vi "Look Up Device Properties.vi"(7 "Lookup Table":string[][](array[string]), 8 "error in (no error)":errorcluster, 9 "Peripheral ID (0)":i32, 10 "Device ID":i32) -> (0 "error out":errorcluster, 1 "Microstep Size":dbl format="%#_6f", 2 "Device Name":string, 5 "Motion Type":string)   [LabVIEW 2018, in "Zaber A Series.lvlib"]
doc: "This VI assists with looking up instrument properties in a table provided by Zaber. You can obtain the device ID and peripheral ID (if applicable) numbers from the device with the Get Device IDs VI, and use the LabVIEW Read Delimited Spreadsheet VI to load the lookup table. Given those inputs, this VI will attempt to find the device position scale factor and its name and motion type.\n\nA prepared table and a Python script for updating it are provided via Zaber's website: https://www.zaber.com/wiki/Software/ASCII_Labview_Driver\n\nNote that this VI is not optimized for speed; for efficiency, do not look up device properties inside high-speed loops.\n\nErrors are produced if the table does not have the expected format, or if the device is not found in the table."
uses:
  Zaber A Series.lvlib
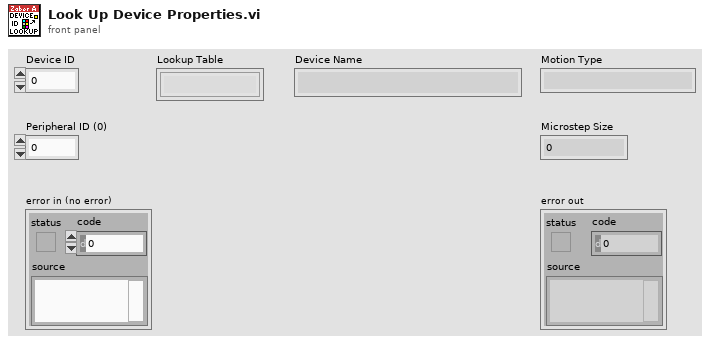
[diagram p1: front panel]
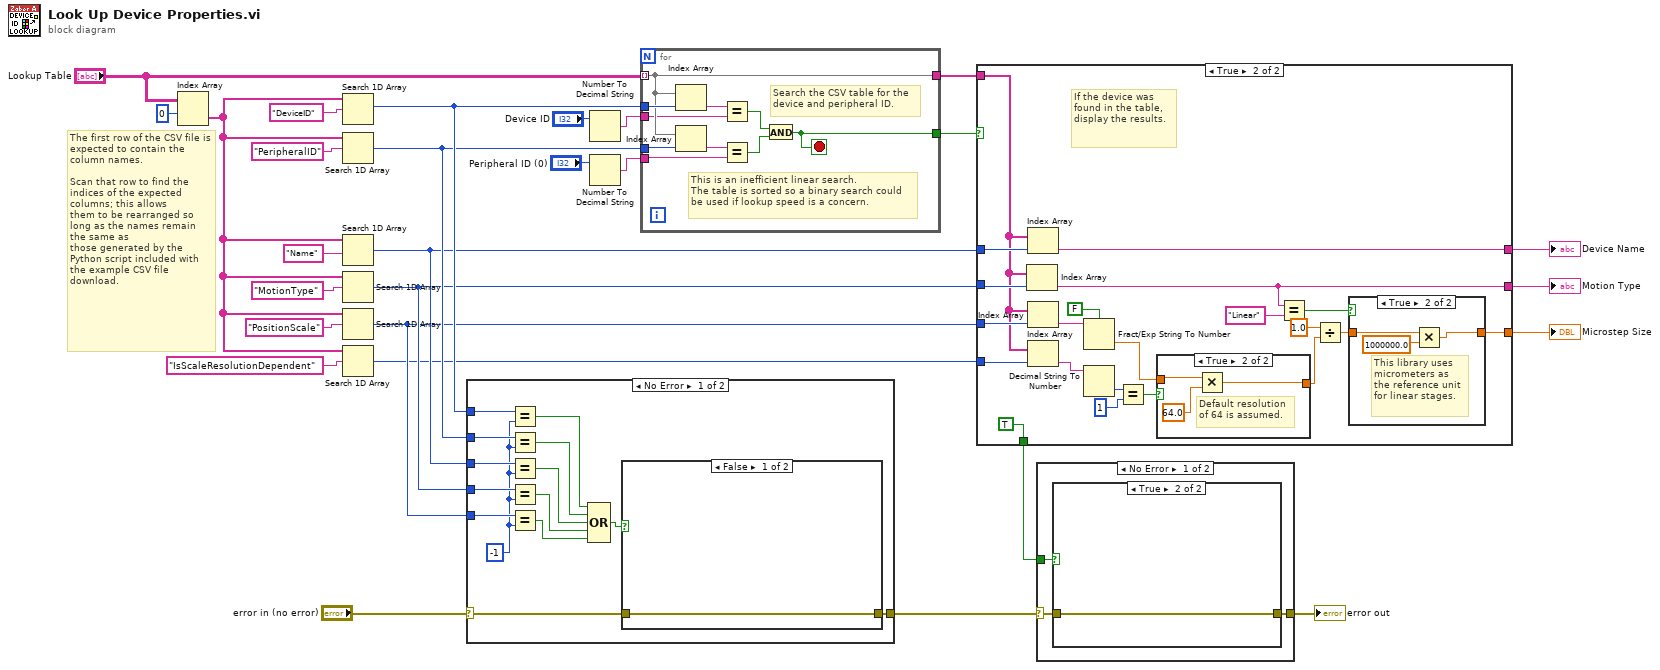
[diagram p0: block diagram]
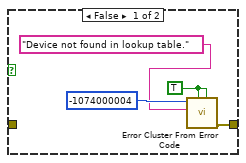
[diagram p2: hidden frame]
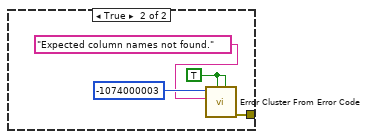
[diagram p4: hidden frame]
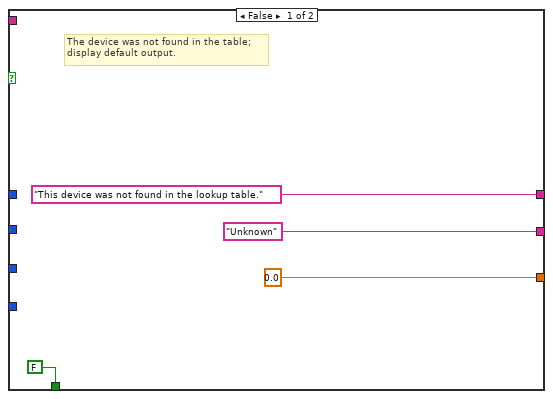
[diagram p6: hidden frame]
diagram:
  # "The first row of the CSV file is expected to contain the column names.\n\nScan that row to find the indices of the expected columns; this allows\nthem to be rearranged so long as the names remain the same as\nthose generated by the Python script included with the example CSV file download."
  n1 = Index Array(array="Lookup Table", index (row)=0) -> (element=w3:string[])  [unwired: 1 in]
  n2 = Search 1D Array(1D array=w3, element="DeviceID") -> (index of element=w16:i32)  [unwired: 1 in]
  n3 = Search 1D Array(1D array=w3, element="PeripheralID") -> (index of element=w15:i32)  [unwired: 1 in]
  n4 = Search 1D Array(1D array=w3, element="Name") -> (index of element=w14:i32)  [unwired: 1 in]
  n5 = Search 1D Array(1D array=w3, element="MotionType") -> (index of element=w13:i32)  [unwired: 1 in]
  n6 = Search 1D Array(1D array=w3, element="PositionScale") -> (index of element=w12:i32)  [unwired: 1 in]
  n7 = Search 1D Array(1D array=w3, element="IsScaleResolutionDependent") -> (index of element=w1:i32)  [unwired: 1 in]
  n8 = case shown="No Error" "error in (no error)" {
    selector: "error in (no error)" -> [w30 w48]
    tunnel: [w32 w48] -> w10
    tunnel: w16 -> [w42 _]
    tunnel: w15 -> [w41 _]
    tunnel: w14 -> [w40 _]
    tunnel: w13 -> [w39 _]
    tunnel: w12 -> [w38 _]
    frame No Error {
      w29 = -1
      n9 = Equal?(x=w42, y=w29) -> (x = y?=w37:bool)
      n10 = Equal?(x=w41, y=w29) -> (x = y?=w36:bool)
      n11 = Equal?(x=w40, y=w29) -> (x = y?=w35:bool)
      n12 = Equal?(x=w39, y=w29) -> (x = y?=w34:bool)
      n13 = Equal?(x=w38, y=w29) -> (x = y?=w33:bool)
      n14 = Compound Arithmetic op=OR(w37, w36, w35, w34, w33) -> (w31:bool)
      n15 = case shown="False" w31 {
        tunnel: [w43 w47] -> w32
        tunnel: w30 -> [w43 _]
        frame False {
        }
        frame True {
          w44 = TRUE ("show call chain? (False)")
          n16 = call <vilib>:"Error Cluster From Error Code.vi"("is warning? (False)"=w44, "show call chain? (False)"=w44, "error message (\"\")"="Expected column names not found." ("error message (\"\")"), "error code (0)"=-1074000003) -> ("error out"=w47:errorcluster)  [unwired: 5 in]
        }
      }
    }
    frame Error {
    }
  }
  n17 = Number To Decimal String(number="Device ID") -> (decimal integer string=w8:string)  [unwired: 1 in]
  n18 = Number To Decimal String(number="Peripheral ID (0)") -> (decimal integer string=w7:string)  [unwired: 1 in]
  n19 = for {
    tunnel: "Lookup Table" -> [w54] mode=indexing
    tunnel: w16 -> [w58]
    tunnel: w15 -> [w57]
    tunnel: w8 -> [w51]
    tunnel: w7 -> [w49]
    tunnel: [w54] -> w19
    tunnel: [w53] -> w23
    stop <- w53 stop-if-true
    # "This is an inefficient linear search.\nThe table is sorted so a binary search could\nbe used if lookup speed is a concern."
    # "Search the CSV table for the\ndevice and peripheral ID."
    n20 = Index Array(array=w54, index=w58) -> (element=w52:string)
    n21 = Index Array(array=w54, index=w57) -> (element=w50:string)
    n22 = Equal?(x=w52, y=w51) -> (x = y?=w56:bool)
    n23 = Equal?(x=w50, y=w49) -> (x = y?=w55:bool)
    n24 = And(x=w56, y=w55) -> (x .and. y?=w53:bool)
  }
  n25 = case shown="True" w23 {
    tunnel: ["This device was not found in the lookup table." w82] -> w22
    tunnel: ["Unknown" w75] -> w21
    tunnel: [0.0 w71] -> w20
    tunnel: w19 -> [_ w70]
    tunnel: w14 -> [_ w83]
    tunnel: w13 -> [_ w81]
    tunnel: w12 -> [_ w80]
    tunnel: [FALSE TRUE] -> w11
    tunnel: w1 -> [_ w69]
    frame False {
      # "The device was not found in the table;\ndisplay default output."
    }
    frame True {
      # "If the device was found in the table, display the results."
      n26 = Index Array(array=w70, index=w81) -> (element=w75:string)
      n27 = Index Array(array=w70, index=w83) -> (element=w82:string)
      n28 = Index Array(array=w70, index=w80) -> (element=w79:string)
      n29 = Index Array(array=w70, index=w69) -> (element=w68:string)
      n30 = Fract/Exp String To Number(use system decimal point (T)=FALSE, string=w79) -> (number=w64:dbl)  [unwired: 2 in, 1 out]
      n31 = Decimal String To Number(string=w68) -> (number=w67:i32)  [unwired: 2 in, 1 out]
      n32 = Equal?(x=w67, y=1) -> (x = y?=w65:bool)
      n33 = case shown="True" w65 {
        tunnel: w64 -> [w84 w86]
        tunnel: [w84 w87] -> w63
        frame False {
        }
        frame True {
          # "Default resolution\nof 64 is assumed."
          n34 = Multiply(x=w86, y=64.0) -> (x*y=w87:dbl)
        }
      }
      n35 = Equal?(x=w75, y="Linear") -> (x = y?=w73:bool)
      n36 = Divide(x=1.0, y=w63) -> (x/y=w72:dbl)
      n37 = case shown="True" w73 {
        tunnel: w72 -> [w88 w91]
        tunnel: [w88 w90] -> w71
        frame False {
        }
        frame True {
          # "This library uses\nmicrometers as\nthe reference unit\nfor linear stages."
          n38 = Multiply(x=w91, y=1000000.0) -> (x*y=w90:dbl)
        }
      }
    }
  }
  "Device Name" <- w22
  "Motion Type" <- w21
  "Microstep Size" <- w20
  n39 = case shown="No Error" w10 {
    selector: w10 -> [w92 w100]
    tunnel: w11 -> [w94 _]
    tunnel: [w93 w100] -> w9
    frame No Error {
      n40 = case shown="True" w94 {
        tunnel: [w96 w99] -> w93
        tunnel: w92 -> [_ w99]
        frame False {
          w95 = TRUE ("show call chain? (False)")
          n41 = call <vilib>:"Error Cluster From Error Code.vi"("is warning? (False)"=w95, "show call chain? (False)"=w95, "error message (\"\")"="Device not found in lookup table." ("error message (\"\")"), "error code (0)"=-1074000004) -> ("error out"=w96:errorcluster)  [unwired: 5 in]
        }
        frame True {
        }
      }
    }
    frame Error {
    }
  }
  "error out" <- w9
